vi "RegisterVI.vi"(8 "error in":errorcluster, 10 "VI Ref":refnum<vi>) -> (0 "error out":errorcluster, 1 "Current Language":string)   [LabVIEW 2017, in "JKI Simple Localization.lvlib"]
doc: "Register a VI to the localizer's registry. Automatically applies the current language to this VI."
uses:
  API/JKI Simple Localization.lvlib
  Definitions/Translation.Action.ctl
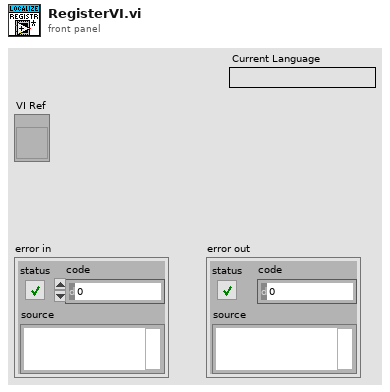
[diagram p1: front panel]
types:
  T1 = typedef "JKI Simple Localization.lvlib/Translation.Action.ctl" = enum16{"Read Dictionary", "Translate VIs", "Register VI", "Get Languages", "Translate Phrase", "Translate VI", "Unregister"}
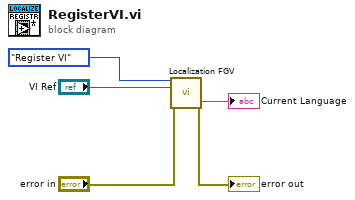
[diagram p0: block diagram]
diagram:
  n1 = call "Localization FGV.vi"("Action"=Translation.Action."Register VI", "VI in"="VI Ref", "error in"="error in") -> ("Current Language"=→"Current Language":string, "error out"=→"error out":errorcluster)  [unwired: 8 in, 3 out]
